vi "Custom errors handler-UI.vi"(9 "Next State":T1, 11 "code":i32) -> ()   [LabVIEW 2020]
uses:
  Typedefs/Top level VI states.ctl
  User Interface/Typedefs/Next state queue data.ctl
  Typedefs/Start-Stop Enum.ctl
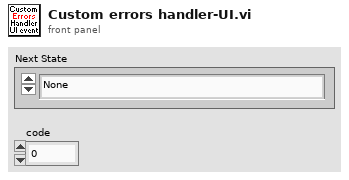
[diagram p1: front panel]
types:
  T1 = typedef "Top level VI states.ctl" = enum16{"None", "Initialise UI", "<STACK PROTOCOL STATES>", "AOL Zstack-START", "AOL Zstack-STOP", "Motor Zstack-START", "Motor Zstack-STOP", "<ACQUISITION PROTOCOL STATES> ", "Functional Acquisition-START", "Functional Acquisition-STOP", "Single Plane Acquisition-START", "Single Plane Acquisition-STOP", "Volume Acquisition-START", "Volume Acquisition-STOP", "<LIVE IMAGING PROTOCOL STATES>", "Live Imaging-START", "Live Imaging-STOP", "Live Plane Imaging-START", "Live Plane Imaging-STOP", "Live Volume Imaging-START", "Live Volume Imaging-STOP", "<MOVEMENT CORRECTION PROTOCOL STATES>", "EXIT"}
  T2 = typedef "Next state queue data.ctl" = cluster{"Start/Stop":T3, "State":T1}
  T3 = typedef "Start-Stop Enum.ctl" = enum16{"START", "STOP"}
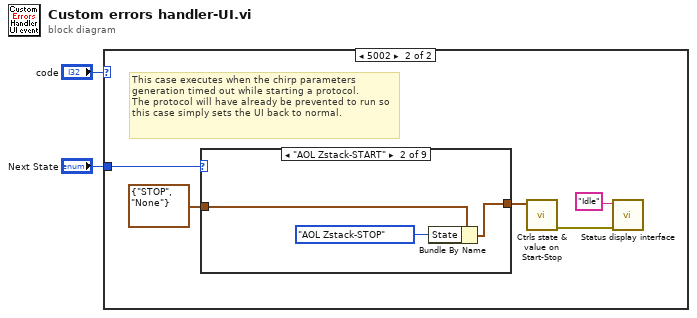
[diagram p0: block diagram]
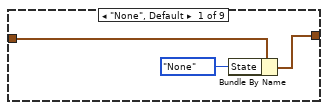
[diagram p3: hidden frame]
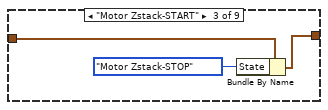
[diagram p4: hidden frame]
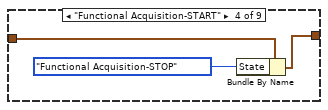
[diagram p5: hidden frame]
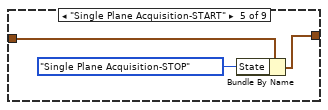
[diagram p6: hidden frame]
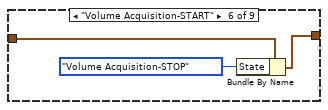
[diagram p7: hidden frame]
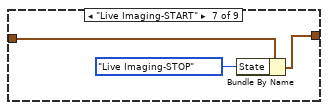
[diagram p8: hidden frame]
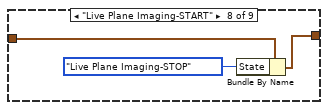
[diagram p9: hidden frame]
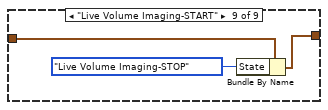
[diagram p10: hidden frame]
diagram:
  n1 = case shown="5002" "code" {
    tunnel: "Next State" -> [_ w5]
    frame 0, Default {
    }
    frame 5002 {
      # "This case executes when the chirp parameters generation timed out while starting a protocol.\nThe protocol will have already be prevented to run so this case simply sets the UI back to normal."
      n2 = case shown="\"AOL Zstack-START\"" w5 {
        tunnel: T2 {"Start/Stop"=enum."STOP", "State"=enum."None"} ("Queue data") -> [w10 w13 w16 w19 w22 w25 w28 w31 w34]
        tunnel: [w8 w11 w14 w17 w20 w23 w26 w29 w32] -> w6
        frame "None", Default {
          n3 = Bundle By Name(cluster=w10, "State"=Top_level_VI_states."None") -> (w8:T2)
        }
        frame "AOL Zstack-START" {
          n4 = Bundle By Name(cluster=w13, "State"=Top_level_VI_states."AOL Zstack-STOP") -> (w11:T2)
        }
        frame "Motor Zstack-START" {
          n5 = Bundle By Name(cluster=w16, "State"=Top_level_VI_states."Motor Zstack-STOP") -> (w14:T2)
        }
        frame "Functional Acquisition-START" {
          n6 = Bundle By Name(cluster=w19, "State"=Top_level_VI_states."Functional Acquisition-STOP") -> (w17:T2)
        }
        frame "Single Plane Acquisition-START" {
          n7 = Bundle By Name(cluster=w22, "State"=Top_level_VI_states."Single Plane Acquisition-STOP") -> (w20:T2)
        }
        frame "Volume Acquisition-START" {
          n8 = Bundle By Name(cluster=w25, "State"=Top_level_VI_states."Volume Acquisition-STOP") -> (w23:T2)
        }
        frame "Live Imaging-START" {
          n9 = Bundle By Name(cluster=w28, "State"=Top_level_VI_states."Live Imaging-STOP") -> (w26:T2)
        }
        frame "Live Plane Imaging-START" {
          n10 = Bundle By Name(cluster=w31, "State"=Top_level_VI_states."Live Plane Imaging-STOP") -> (w29:T2)
        }
        frame "Live Volume Imaging-START" {
          n11 = Bundle By Name(cluster=w34, "State"=Top_level_VI_states."Live Volume Imaging-STOP") -> (w32:T2)
        }
      }
      n12 = call "Ctrls state & value on Start-Stop.vi"("Queue data"=w6) -> ("error out"=w3:errorcluster)  [unwired: 10 in]
      n13 = call "Status display interface.vi"("error in (no error)"=w3, "Message"="Idle") -> ()  [unwired: 9 in, 1 out]
    }
  }
